vi "RES Get Max value.vi"(11 "Table in":refnum<vi>) -> ()   [LabVIEW 2020]
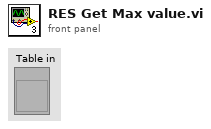
[diagram p1: front panel]
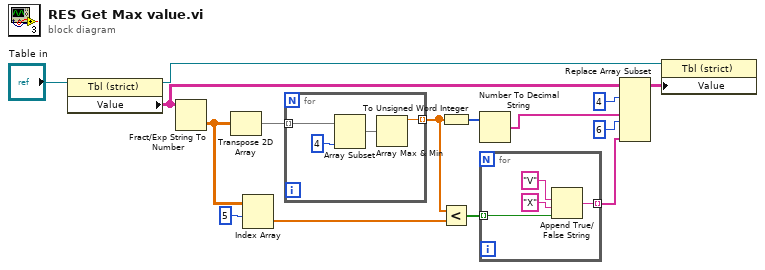
[diagram p0: block diagram]
diagram:
  n1 = property class="Tbl (strict)"(reference="Table in") -> (reference out=w13:refnum<vi>, "Value"=w12:string[][])  [unwired: 1 in, 1 out]
  n2 = Fract/Exp String To Number(string=w12) -> (number=w7:dbl[][])  [unwired: 3 in, 1 out]
  n3 = Transpose 2D Array(2D array=w7) -> (transposed array=w14:dbl[][])
  n4 = Index Array(array=w7, index (row)=5 ("length")) -> (element=w5:dbl[])  [unwired: 1 in]
  n5 = for {
    tunnel: w14 -> [w19] mode=indexing
    tunnel: [w16] -> w6 mode=indexing
    n6 = Array Subset(array=w19, length=4) -> (w17:dbl[])  [unwired: 1 in]
    n7 = Array Max & Min(array=w17) -> (max value=w16:dbl)  [unwired: 3 out]
  }
  n8 = To Unsigned Word Integer(number=w6) -> (unsigned 16bit integer=w8:u16[])
  n9 = Less?(x=w6, y=w5) -> (x < y?=w4:bool[])
  n10 = Number To Decimal String(number=w8) -> (decimal integer string=w9:string[])  [unwired: 1 in]
  n11 = for {
    tunnel: w4 -> [w23] mode=indexing
    tunnel: [w20] -> w2 mode=indexing
    n12 = Append True/False String(1:w23, 2:"X" ("true string"), 3:"V" ("true string")) -> (0:w20:string)  [unwired: 1 in]
  }
  n13 = Replace Array Subset(array=w12, new element #1=w9, index (row) #1=4 ("index (row)"), new element #2=w2, index (row) #2=6 ("index (row)")) -> (w11:string[][])  [unwired: 2 in]
  n14 = property class="Tbl (strict)"(reference=w13, "Value"=w11) -> ()  [unwired: 1 in, 2 out]
